vi "Sim_Wrist.vi"(6 "Battery Voltage":dbl=12.0 format="%#_13g", 9 "StartPoseDegrees":dbl, 11 "Motor1 Dmd":dbl) -> (0 "Motor Current":dbl, 1 "AtLowLimit":bool, 2 "At HIgh LImit":bool, 3 "WritstPositionDegrees":dbl)   [LabVIEW 2023]
uses:
  <vilib>/Rock Robotics/WPI/ThirdParty/JAS_Junk/TrajLib/Enum/DCMOTOR_TYPES_ENUM.ctl
  Robot Global Data.vi
  <vilib>/Rock Robotics/WPI/ThirdParty/JAS_Junk/TrajLib/Trajectory_Library.lvlib
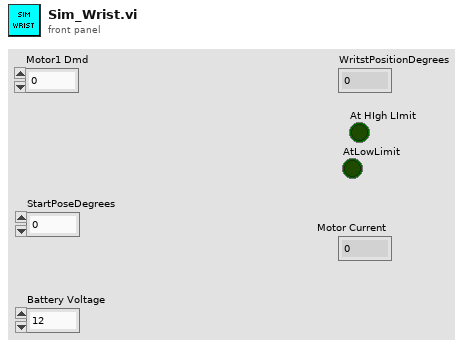
[diagram p1: front panel]
types:
  T1 = typedef "Trajectory_Library.lvlib/DCMOTOR_TYPES_ENUM.ctl" = enum16{"CIM", "AndyMark 9015", "Andy Mark RS 775 125", "Bag", "BaneBots RS 550", "BaneBots RS 775", "Falcon 500", "Mini CIM", "NEO", "NEO 550", "Romi BuiltIn", "Vex 775 Pro", "Snow Blower AM 2235A", "Bosch Seat AM 3493", "Falcon 500 FOC", "Kraken X60", "Kraken X60 FOC", "NEO Vortex"}
  T2 = typedef "Trajectory_Library.lvlib/LINEAR_SYSTEM_ID_SINGLE_JOINT_ARM_MODEL.ctl" = cluster{"DCMOTOR_TYPES":T1, "Num Motors":i32, "ArmLength_M":dbl, "massKg":dbl, "Gearing":dbl, "MOI kgm2":dbl, "Estimate MOI":bool}
  T3 = typedef "Trajectory_Library.lvlib/SINGLE_JOINT_ARM_SIM_SIMULATION_PARAMS.ctl" = cluster{"MinAngle_Rad":dbl, "MaxAngle_Rad":dbl, "Measurment StdDev":dbl, "SimulateGravity":bool}
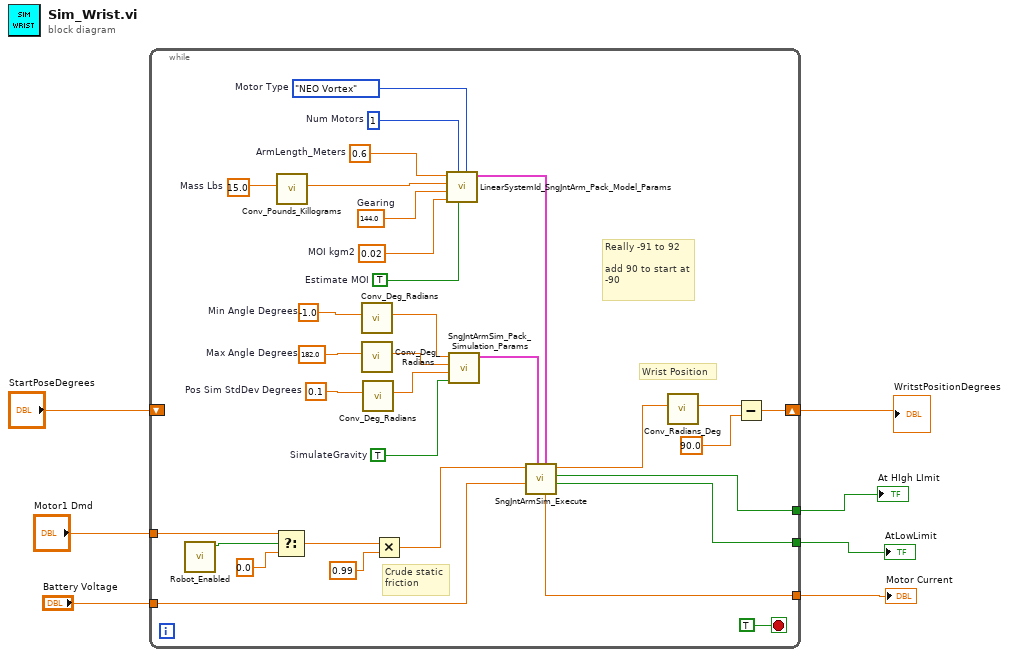
[diagram p0: block diagram]
diagram:
  n1 = while {
    shift-right: [w14] -> w6
    shift-left: "StartPoseDegrees" -> [_]
    tunnel: "Battery Voltage" -> [w15]
    tunnel: [w27] -> w4
    tunnel: [w26] -> w3
    tunnel: [w16] -> w2
    tunnel: "Motor1 Dmd" -> [w11]
    stop <- TRUE stop-if-true
    w31 = TRUE  # Estimate MOI
    w32 = 0.02  # MOI kgm2
    w22 = -1.0  # Min Angle Degrees
    w23 = 182.0  # Max Angle Degrees
    w24 = 0.1  # Pos Sim StdDev Degrees
    w33 = TRUE  # SimulateGravity
    w34 = 0.6  # ArmLength_Meters
    w35 = 144.0  # Gearing
    w18 = 15.0  # Mass Lbs
    w36 = 1  # Num Motors
    w37 = DCMOTOR_TYPES_ENUM."NEO Vortex"  # Motor Type
    # "Really -91 to 92\n\nadd 90 to start at\n-90"
    # "Wrist Position"
    # "Crude static\nfriction"
    n2 = call "Robot_Enabled.vi"() -> ("Robot Enabled"=w10:bool)  [unwired: 11 in]
    n3 = Select(t=w11, s=w10, f=0.0) -> (s? t:f=w8:dbl)
    n4 = call <vilib>:"Conv_Pounds_Killograms.vi"("Pounds"=w18) -> ("Killograms"=w17:dbl)  [unwired: 10 in]
    n5 = call <vilib>:"Conv_Deg_Radians.vi"("Degress"=w22) -> ("Radians"=w21:dbl)  [unwired: 10 in]
    n6 = call <vilib>:"Conv_Deg_Radians.vi"("Degress"=w23) -> ("Radians"=w20:dbl)  [unwired: 10 in]
    n7 = call <vilib>:"Conv_Deg_Radians.vi"("Degress"=w24) -> ("Radians"=w19:dbl)  [unwired: 10 in]
    n8 = Multiply(x=w8, y=0.99) -> (x*y=w28:dbl)
    n9 = call <vilib>:"LinearSystemId_SngJntArm_Pack_Model_Params.vi"("DCMOTOR_TYPES"=w37, "Estimate MOI"=w31, "Num Motors"=w36, "MOI kgm2"=w32, "Gearing"=w35, "massKg"=w17, "ArmLength_M"=w34) -> ("SngJntArmSim_Model _Params"=w30:T2)  [unwired: 4 in]
    n10 = call <vilib>:"SngJntArmSim_Pack_Simulation_Params.vi"("SimulateGravity"=w33, "Pos Sim StdDev Rad"=w19, "MaxAngle_Rad"=w20, "MinAngle_Rad"=w21) -> ("SngJntArmSim_Simulation _Params"=w29:T3)  [unwired: 7 in]
    n11 = call <vilib>:"SngJntArmSim_Execute.vi"("SngJntArmSim_Model _Params"=w30, "SngJntArmSim_Simulation _Params"=w29, "Battery Volts"=w15, "Motor Dmd"=w28) -> ("AtLowLimit"=w26:bool, "At HIgh LImit"=w27:bool, "ArmAngle_Rad"=w25:dbl, "Motor Current"=w16:dbl)  [unwired: 2 in, 2 out]
    n12 = call <vilib>:"Conv_Radians_Deg.vi"("Radians"=w25) -> ("Degrees"=w13:dbl)  [unwired: 10 in]
    n13 = Subtract(x=w13, y=90.0) -> (x-y=w14:dbl)
  }
  "WritstPositionDegrees" <- w6
  "At HIgh LImit" <- w4
  "AtLowLimit" <- w3
  "Motor Current" <- w2
